vi "Read Coords.vi"(8 "error in (no error)":errorcluster, 11 "ListboxEditCellMsg in":refnum<class "ListboxEditCellMsg.lvclass">) -> (0 "error out":errorcluster, 2 "Coords":T1, 3 "ListboxEditCellMsg out":refnum<class "ListboxEditCellMsg.lvclass">)   [LabVIEW 2015, in "ActorEvents.lvlib" / "ListboxEditCellMsg.lvclass"]
uses:
  ListboxEditCellMsg.lvclass
  <vilib>/Utility/miscctls.llb/LVRowAndColumnTypeDef.ctl
  ListboxEditCellMsg.lvclass/ListboxEditCellMsg.ctl
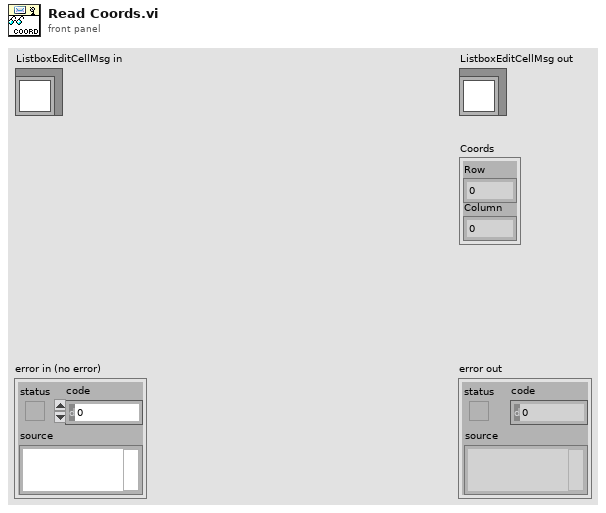
[diagram p1: front panel]
types:
  T1 = typedef "LVRowAndColumnTypeDef.ctl" = cluster{"Row":i32, "Column":i32}
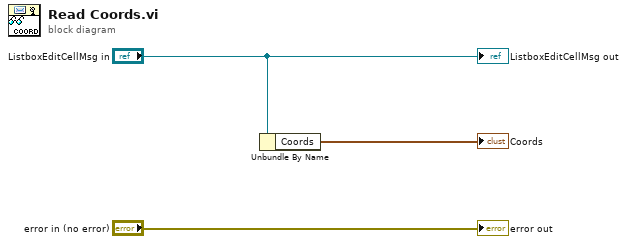
[diagram p0: block diagram]
diagram:
  n1 = Unbundle By Name("ListboxEditCellMsg in") -> ("Coords"=→"Coords":T1)
  "error out" <- "error in (no error)"
  "ListboxEditCellMsg out" <- "ListboxEditCellMsg in"
